vi "Create Coverage Report - Lines is Sum of Nodes and Diagrams.vi"() -> ()   [LabVIEW 2017, in "Cobertura.Tests.lvlib"]
uses:
  Cobertura.Tests.lvlib
  Cobertura/Coverage/Coverage.lvclass/Coverage.ctl
  Cobertura/Package/Package.lvclass/Package.ctl
  Cobertura/Class/Class.lvclass/Class.ctl
  Cobertura/Method/Method.lvclass/Method.ctl
  Cobertura/Coverage/Read Packages.vi
  Cobertura/Package/Read Classes.vi
  Cobertura/Class/Read Methods.vi
  Cobertura/Method/Read Lines.vi
  Fake Project Inspector/Fake Project Inspector.lvclass
  C:/Users/Pascal/Projects/Home/lvunit/Cobertura/Project Inspector Base/Project Inspector Base.lvclass
  Fake Code Coverage/Fake Code Coverage.lvclass
  C:/Users/Pascal/Projects/Home/lvunit/Code Coverage/Code Coverage.lvclass
  Fake Code Inspector/Fake Code Inspector.lvclass
  C:/Users/Pascal/Projects/Home/lvunit/Cobertura/Code Inspector Base/Code Inspector Base.lvclass
  Cobertura/Package/Package.lvclass
  Cobertura/Class/Class.lvclass
  Cobertura/Method/Method.lvclass
  Cobertura/Line/Line.lvclass
  Cobertura/Cobertura.lvlib
  Cobertura/Coverage/Coverage.lvclass
  <vilib>/PNR/Transparent Assertions/Transparent Assertions/Transparent Assertions.lvlib
panel:
  out "error out":errorcluster
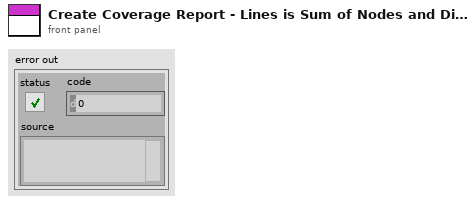
[diagram p1: front panel]
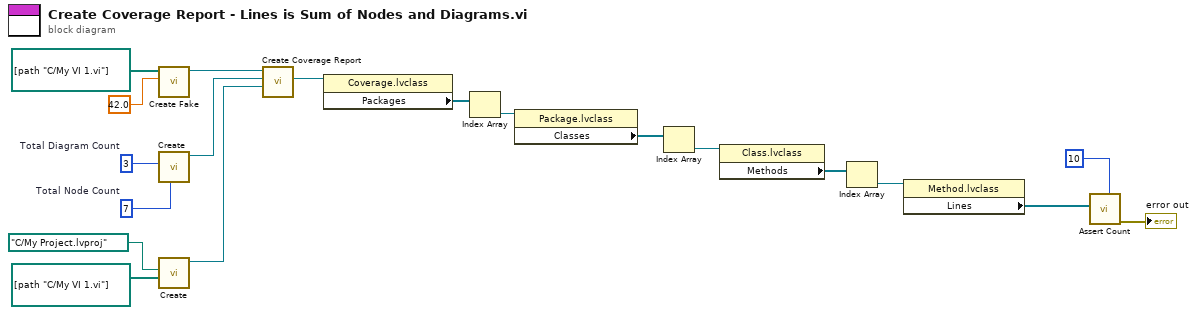
[diagram p0: block diagram]
diagram:
  w1 = 7  # Total Node Count
  w2 = 3  # Total Diagram Count
  n1 = call "Create Fake.vi"("Coverage Percentage"=42.0, "All VIs Measured"=path[] [path "C:/My VI 1.vi"] ("Item Paths")) -> ("Fake Code Coverage"=w7:refnum<class "Fake Code Coverage.lvclass">)  [unwired: 8 in, 1 out]
  n2 = call "Create.vi"("Total Node Count"=w1, "Total Diagram Count"=w2) -> ("Fake Code Inspector"=w3:refnum<class "Fake Code Inspector.lvclass">)  [unwired: 8 in, 1 out]
  n3 = call "Create.vi"("Item Paths"=path[] [path "C:/My VI 1.vi"], "Path"=path "C:/My Project.lvproj") -> ("Fake Project Inspector"=w16:refnum<class "Fake Project Inspector.lvclass">)  [unwired: 8 in, 1 out]
  n4 = call "Create Coverage Report.vi"("Project Inspector"=w16, "Code Inspector"=w3, "CodeCoverage in"=w7) -> ("Coverage"=w19:refnum<class "Coverage.lvclass">)  [unwired: 7 in, 1 out]
  n5 = property class="Coverage.lvclass"(reference=w19) -> ("Packages"=w17:refnum<class "Package.lvclass">[])  [unwired: 1 in, 2 out]
  n6 = Index Array(array=w17) -> (element=w14:refnum<class "Package.lvclass">)  [unwired: 1 in]
  n7 = property class="Package.lvclass"(reference=w14) -> ("Classes"=w13:refnum<class "Class.lvclass">[])  [unwired: 1 in, 2 out]
  n8 = Index Array(array=w13) -> (element=w11:refnum<class "Class.lvclass">)  [unwired: 1 in]
  n9 = property class="Class.lvclass"(reference=w11) -> ("Methods"=w10:refnum<class "Method.lvclass">[])  [unwired: 1 in, 2 out]
  n10 = Index Array(array=w10) -> (element=w9:refnum<class "Method.lvclass">)  [unwired: 1 in]
  n11 = property class="Method.lvclass"(reference=w9) -> ("Lines"=w8:refnum<class "Line.lvclass">[])  [unwired: 1 in, 2 out]
  n12 = call <vilib>:"Assert Count.vi"("Expected"=10 ("Branch Rate"), "Haystack"=w8) -> ("error out"=→"error out":errorcluster)  [unwired: 9 in]
